vi "SSC Digital Configure Time Set Edge.vi"(0 "Digital SSC in":T2[](array[typedef]), 5 "time set":string caption="Time Set", 7 "edge":T1=2800 items=["Drive On"=2800, "Drive Data"=2801, "Drive Return"=2802, "Drive Off"=2803, "Compare Strobe"=2804, "Drive Data 2"=2805, "Drive Return 2"=2806, "Compare Strobe 2"=2807], 9 "time (s)":dbl format="%#_6p", 11 "error in":errorcluster) -> (4 "Digital SSC out":T2[](array[typedef]), 15 "error out":errorcluster)   [LabVIEW 2019]
doc: "Configures the tset edge. \nBelow are the corresponding property from mflex code.\n\n• chEdgeD0: Drive On \n• chEdgeD1: Drive Data \n• chEdgeD2: Drive Return \n• chEdgeD3: Drive Off \n• chEdgeR0: Compare Open \n• chEdgeR1: Compare Close"
uses:
  SSC Digital.ctl
  <instrlib>/niDigital/niDigital.llb/niDigital Time Set Edge Type.ctl
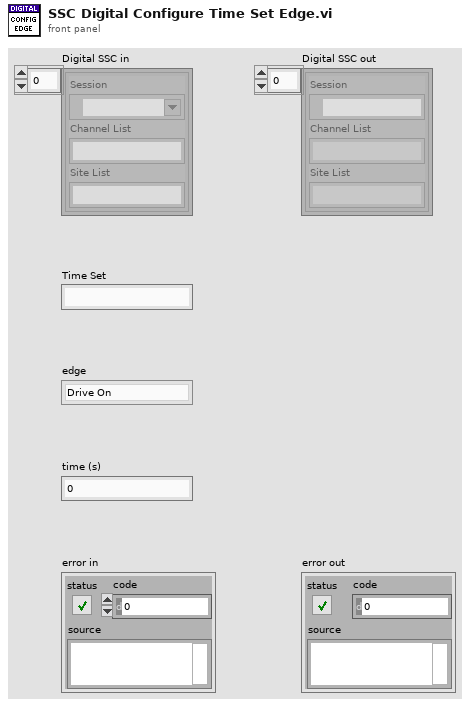
[diagram p1: front panel]
types:
  T1 = typedef "niDigital Time Set Edge Type.ctl" = i32
  T2 = typedef "SSC Digital.ctl" = cluster{"Session":refnum<k15>, "Channel List":string, "Site List":string}
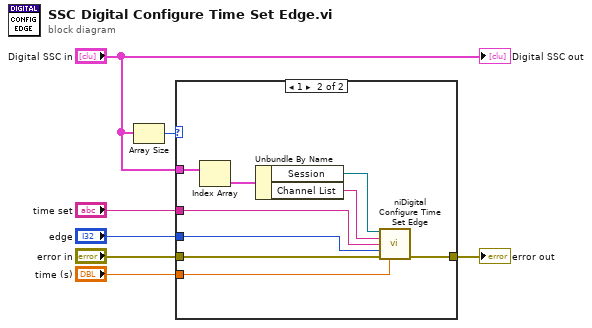
[diagram p0: block diagram]
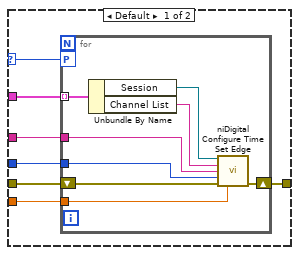
[diagram p2: hidden frame]
diagram:
  n1 = Array Size(array="Digital SSC in") -> (size(s)=w5:i32)
  n2 = case shown="1" w5 {
    selector: w5 -> [w14 _]
    tunnel: "error in" -> [w12 w28]
    tunnel: [w10 w29] -> w6
    tunnel: "Digital SSC in" -> [w13 w31]
    tunnel: "time set" -> [w11 w25]
    tunnel: "edge" -> [w9 w24]
    tunnel: "time (s)" -> [w8 w23]
    frame Default {
      n3 = for {
        workers-P: w14 -> [_]
        tunnel: w13 -> [w22] mode=indexing
        tunnel: w11 -> [w17]
        shift-right: [w20] -> w10
        shift-left: w12 -> [w21]
        tunnel: w9 -> [w16]
        tunnel: w8 -> [w15]
        n4 = Unbundle By Name(w22) -> ("Session"=w19:refnum<k15>, "Channel List"=w18:string)
        n5 = call <instrlib>:"niDigital Configure Time Set Edge.vi"("instrument handle"=w19, "pin list"=w18, "time set"=w17, "edge"=w16, "error in"=w21, "time (s)"=w15) -> ("error out"=w20:errorcluster)  [unwired: 8 in, 1 out]
      }
    }
    frame 1 {
      n6 = Index Array(array=w31) -> (element=w30:T2)  [unwired: 1 in]
      n7 = Unbundle By Name(w30) -> ("Session"=w27:refnum<k15>, "Channel List"=w26:string)
      n8 = call <instrlib>:"niDigital Configure Time Set Edge.vi"("instrument handle"=w27, "pin list"=w26, "time set"=w25, "edge"=w24, "error in"=w28, "time (s)"=w23) -> ("error out"=w29:errorcluster)  [unwired: 8 in, 1 out]
    }
  }
  "error out" <- w6
  "Digital SSC out" <- "Digital SSC in"
